vi "Create a Cell.vi"(8 "error in (no error)":errorcluster, 10 "Run Instance":refnum<class "Run Instance.lvclass">, 11 "Repetitions":u32=1) -> (0 "error out":errorcluster, 3 "Schedule Cell out":refnum<class "Schedule Cell.lvclass">)   [LabVIEW 2020, in "CIRCUS_uServices.lvlib" / "Run Utilities.lvlib" / "Schedule Cell.lvclass"]
doc: "Create a new cell of the provided Run Instance for the duration of the number of Repetitions"
uses:
  Schedule Cell.lvclass
  Run Instance/Run Instance.lvclass
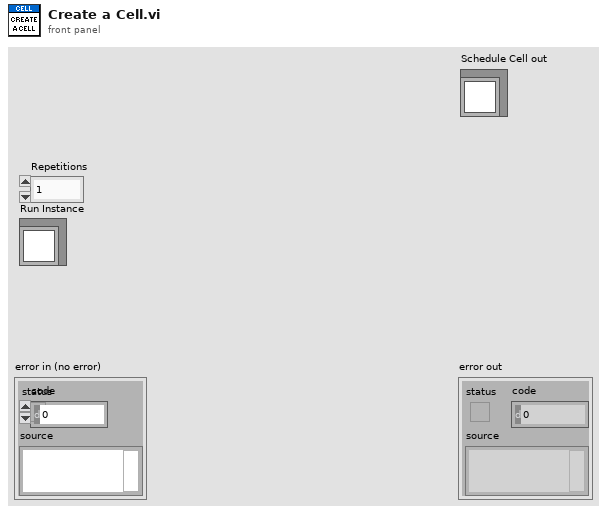
[diagram p1: front panel]
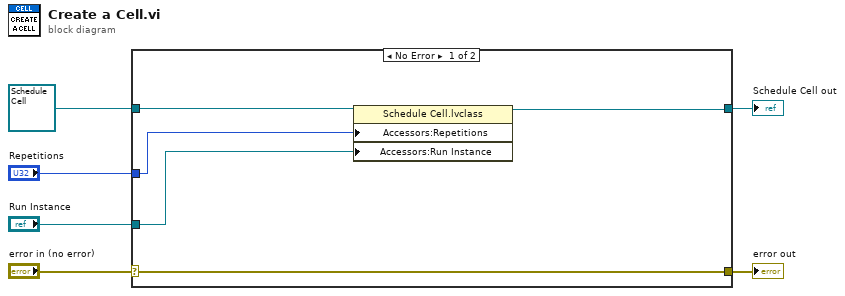
[diagram p0: block diagram]
diagram:
  n1 = case shown="No Error" "error in (no error)" {
    selector: "error in (no error)" -> [w11 w13]
    tunnel: [w11 w13] -> w5
    tunnel: [w9 w12] -> w3
    tunnel: refnum<class "Schedule Cell.lvclass"> refnum ("Schedule Cell in") -> [w10 w12]
    tunnel: "Repetitions" -> [w8 _]
    tunnel: "Run Instance" -> [w7 _]
    frame No Error {
      n2 = property class="Schedule Cell.lvclass"(reference=w10, "Accessors:Repetitions"=w8, "Accessors:Run Instance"=w7) -> (reference out=w9:refnum<class "Schedule Cell.lvclass">)  [unwired: 1 in, 1 out]
    }
    frame Error {
    }
  }
  "error out" <- w5
  "Schedule Cell out" <- w3
